vi "SpreadsheetRead.vi"() -> ()   [LabVIEW 2014]
uses:
  <vilib>/Utility/file.llb/Read From Spreadsheet File (DBL).vi
panel:
  out "Column 0":dbl[](array[numeric])
  out "Column 1":dbl[](array[numeric])
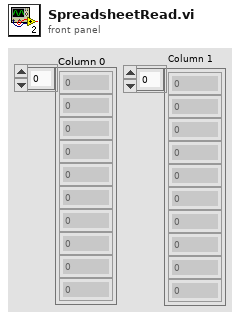
[diagram p1: front panel]
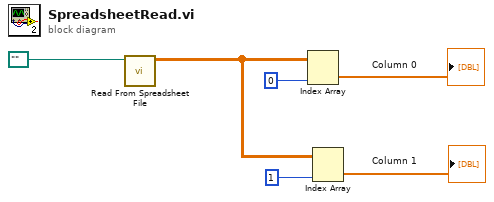
[diagram p0: block diagram]
diagram:
  n1 = call-poly <vilib>:"Read From Spreadsheet File.vi"("file path (dialog if empty)"=path "") -> ("all rows"=w4:dbl[][])  [unwired: 6 in, 4 out]
  n2 = Index Array(array=w4, index (col)=0 ("disabled index (col)")) -> (element=→"Column 0":dbl[])  [unwired: 1 in]
  n3 = Index Array(array=w4, index (col)=1 ("disabled index (col)")) -> (element=→"Column 1":dbl[])  [unwired: 1 in]
